vi "19.6-DirectIIR-SinglePole-LP.vi"() -> ()   [LabVIEW 2020]
doc: "Uses the Median Filter VI to analyze pulses in the presence of noise. The example generates a pulse contaminated with Gaussian noise and applies a median filter. For comparison purposes, the VI computes the pulse parameters of the filtered pulse."
uses:
  <vilib>/Analysis/3filter.llb/IIR Filter (DBL).vi
  <vilib>/Analysis/NI_AALBase.lvlib
panel:
  in  "stop":bool
  out "p":dbl format="%.2f"
  out "Sig":dbl[](graph)
  out "H[k] 2":dbl[](graph)
  in  "Fc":dbl(slide)=25.974025974025974 scale=0.0..400.0
  in  "Fs":dbl(slide)=1024.0 scale=800.0..1024.0
  out "Filtered2":dbl[](graph)
  out "Filtered1":dbl[](graph)
  out "H[k]1":dbl[](graph)
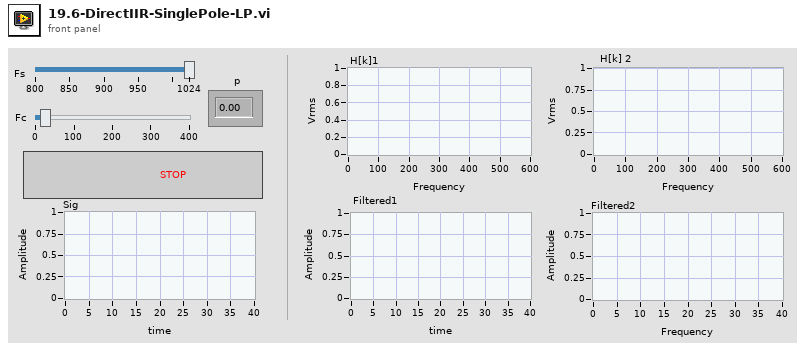
[diagram p1: front panel]
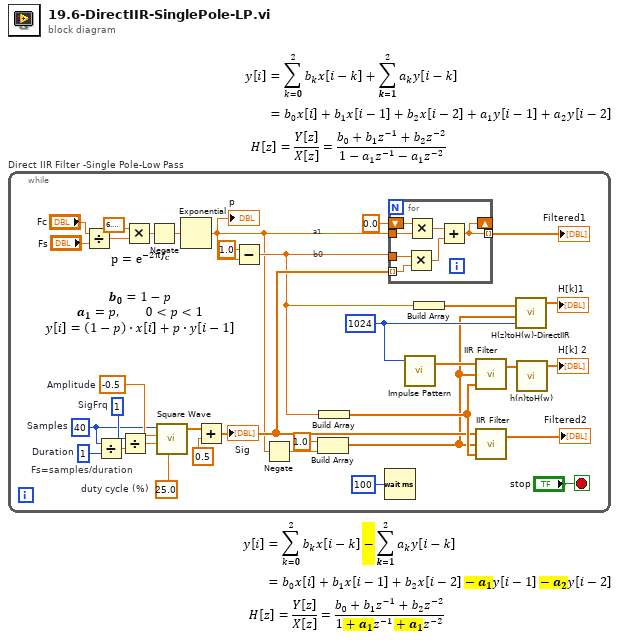
[diagram p0: block diagram]
diagram:
  n1 = while "Direct IIR Filter -Single Pole-Low Pass" {
    stop <- "stop" stop-if-true
    w7 = 1  # Duration
    w11 = 1024 ("FFT size")
    w27 = 1  # SigFrq
    w28 = 25.0  # duty cycle (%)
    w29 = -0.5  # Amplitude
    w9 = 40  # Samples
    # "b0"
    # "a1"
    # "Fs=samples/duration"
    n2 = Divide(x="Fc", y="Fs") -> (x/y=w22:dbl)
    n3 = Divide(x=w9, y=w7) -> (x/y=w8:dbl)
    n4 = Divide(x=w27, y=w8) -> (x/y=w23:dbl)
    n5 = Multiply(x=6.283185307179586, y=w22) -> (x*y=w31:dbl)
    n6 = Negate(x=w31) -> (-x=w30:dbl)
    n7 = call <vilib>:"Square Wave.vi"("samples"=w9, "amplitude"=w29, "frequency"=w23, "duty cycle (%)"=w28) -> ("square wave"=w25:dbl[])  [unwired: 2 in, 2 out]
    n8 = Exponential(1:w30) -> (0:w4:dbl)
    "p" <- w4
    n9 = Add(x=w25, y=0.5) -> (x+y=w10:dbl[])
    "Sig" <- w10
    n10 = Subtract(x=1.0, y=w4) -> (x-y=w6:dbl)
    n11 = Negate(x=w4) -> (-x=w12:dbl)
    n12 = Build Array(1.0 ("element"), w12) -> (w1:dbl[])
    n13 = Build Array(w6) -> (w18:dbl[])
    n14 = Wait (ms)(milliseconds to wait=u32 100) -> ()  [unwired: 1 out]
    n15 = for {
      tunnel: w10 -> [w38] mode=indexing
      shift-right: [w35] -> _
      shift-left: 0.0 -> [w41]
      tunnel: w4 -> [w40]
      tunnel: w6 -> [w39]
      tunnel: [w35] -> w15 mode=indexing
      n16 = Multiply(x=w39, y=w38) -> (x*y=w37:dbl)
      n17 = Multiply(x=w41, y=w40) -> (x*y=w36:dbl)
      n18 = Add(x=w36, y=w37) -> (x+y=w35:dbl)
    }
    "Filtered1" <- w15
    n19 = call <vilib>:"Impulse Pattern.vi"("samples"=w11) -> ("Impulse Pattern"=w19:dbl[])  [unwired: 2 in, 1 out]
    n20 = Build Array(w6) -> (w21:dbl[])
    n21 = call-poly <vilib>:"IIR Filter.vi"("Forward Coefficients"=w18, "Reverse Coefficients"=w1, "X"=w19) -> ("Filtered X"=w16:dbl[])  [unwired: 1 in, 1 out]
    n22 = call-poly <vilib>:"IIR Filter.vi"("Forward Coefficients"=w18, "Reverse Coefficients"=w1, "X"=w10) -> ("Filtered X"=→"Filtered2":dbl[])  [unwired: 1 in, 1 out]
    n23 = call "H(z)toH(w)-DirectIIR.vi"("FFT size"=w11, "Reverse"=w1, "Forward"=w21) -> ("Mag H(w)"=→"H[k]1":dbl[])  [unwired: 2 out]
    n24 = call "h(n)toH(w).vi"("h(n)"=w16) -> ("Mag H(w)"=→"H[k] 2":dbl[])  [unwired: 1 in, 2 out]
  }
